vi "Read Last RRG Conf.vi"() -> (10 "max2":sgl, 11 "description 2":string, 12 "max1":sgl, 13 "description 1":string, 14 "s2":dbl, 15 "s1":dbl, 16 "ind2":dbl, 17 "ind1":dbl, 18 "rrg2":T1, 19 "rrg1":T1)   [LabVIEW 2020]
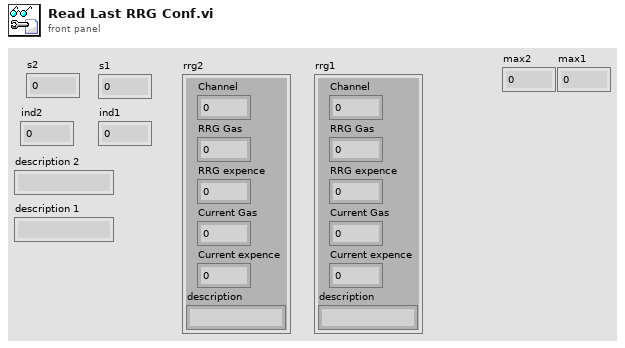
[diagram p1: front panel]
types:
  T1 = cluster{"Channel":i32, "RRG Gas":sgl, "RRG expence":sgl, "Current Gas":sgl, "Current expence":sgl, "description":string}
  T2 = cluster{"s2":dbl, "s1":dbl, "ind2":dbl, "ind1":dbl, "rrg2":cluster{"Channel":i32, "RRG Gas":sgl, "RRG expence":sgl, "Current Gas":sgl, "Current expence":sgl, "description":string}, "rrg1":cluster{"Channel":i32, "RRG Gas":sgl, "RRG expence":sgl, "Current Gas":sgl, "Current expence":sgl, "description":string}}
  T3 = enum16{"open", "replace", "create", "open or create", "replace or create", "replace or create with confirmation"}
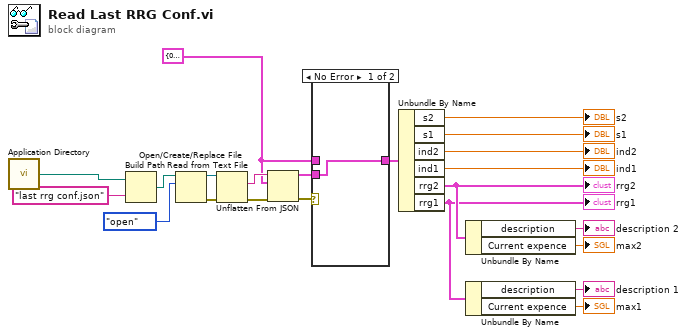
[diagram p0: block diagram]
diagram:
  w12 = T2 {"s2"=0.0, "s1"=0.0, "ind2"=0.0, "ind1"=0.0, "rrg2"={"Channel"=2, "RRG Gas"=0.0, "RRG expence"=0.0, "Current Gas"=0.0, "Current expence"=0.0, "description"="Не выбрано"}, "rrg1"={"Channel"=1, "RRG Gas"=0.0, "RRG expence"=0.0, "Current Gas"=0.0, "Current expence"=0.0, "description"="Не выбрано"}}
  n1 = call <vilib>:"Application Directory.vi"() -> ("Application Directory"=w22:path)
  n2 = Build Path(base path=w22, name or relative path="last rrg conf.json") -> (appended path=w20:path)
  n3 = Open/Create/Replace File(file path (use dialog)=w20, operation (0:open)=T3."open") -> (refnum out=w16:refnum<file>, error out=w15:errorcluster)  [unwired: 4 in, 1 out]
  n4 = Read from Text File(file (use dialog)=w16, error in=w15) -> (text=w17:string, error out=w18:errorcluster)  [unwired: 2 in, 2 out]
  n5 = Unflatten From JSON(JSON string=w17, type and defaults=w12, error in (no error)=w18) -> (value=w13:T2, error out=w14:errorcluster)  [unwired: 4 in]
  n6 = case shown="No Error" w14 {
    tunnel: w13 -> [w23 _]
    tunnel: w12 -> [_ w24]
    tunnel: [w23 w24] -> w11
    frame No Error {
    }
    frame Error {
    }
  }
  n7 = Unbundle By Name(w11) -> ("s2"=→"s2":dbl, "s1"=→"s1":dbl, "ind2"=→"ind2":dbl, "ind1"=→"ind1":dbl, "rrg2"=w6:T1, "rrg1"=w3:T1)
  "rrg2" <- w6
  "rrg1" <- w3
  n8 = Unbundle By Name(w6) -> ("description"=→"description 2":string, "Current expence"=→"max2":sgl)
  n9 = Unbundle By Name(w3) -> ("description"=→"description 1":string, "Current expence"=→"max1":sgl)
